vi "Read Result Data.vi"(8 "error in (no error)":errorcluster, 11 "HGF_DataAnalysis in":refnum<class "HGF_DataAnalysis.lvclass">) -> (0 "error out":errorcluster, 2 "Result Data":refnum<class "HGF_VariantDataObject.lvclass">, 3 "HGF_DataAnalysis out":refnum<class "HGF_DataAnalysis.lvclass">)   [LabVIEW 2012, in "HGF_DataAnalyzer.lvlib" / "HGF_DataAnalysis.lvclass"]
uses:
  HGF_DataAnalysis.lvclass
  HGF_LVC/HGF_BaseClasses/HGF_VariantDataObject/HGF_VariantDataObject.lvclass
  HGF_DataAnalysis.lvclass/HGF_DataAnalysis.ctl
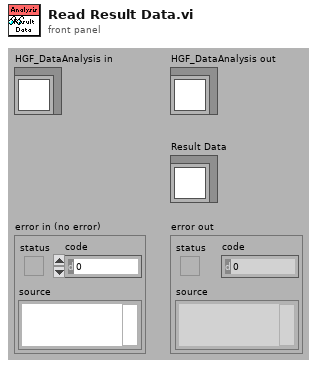
[diagram p1: front panel]
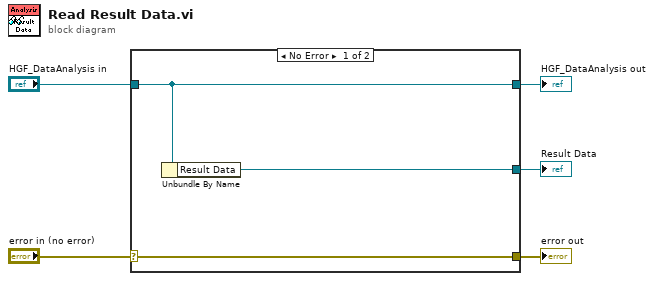
[diagram p0: block diagram]
diagram:
  n1 = case shown="No Error" "error in (no error)" {
    selector: "error in (no error)" -> [w8 w9]
    tunnel: [w8 w9] -> w4
    tunnel: [w7 w10] -> w2
    tunnel: "HGF_DataAnalysis in" -> [w7 w10]
    tunnel: [w6 _] -> w1
    frame No Error {
      n2 = Unbundle By Name(w7) -> ("Result Data"=w6:refnum<class "HGF_VariantDataObject.lvclass">)
    }
    frame Error {
    }
  }
  "error out" <- w4
  "HGF_DataAnalysis out" <- w2
  "Result Data" <- w1
